vi "Extract CMD_Data.vi"(11 "Frame":string) -> (1 "DATA":string, 2 "Status":string, 3 "CMD":string)   [LabVIEW 2020, in "Library Test.lvlib" / "P2056_Send_Command_UART.lvclass"]
uses:
  P2056_Send_Command_UART.lvclass
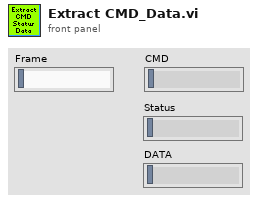
[diagram p1: front panel]
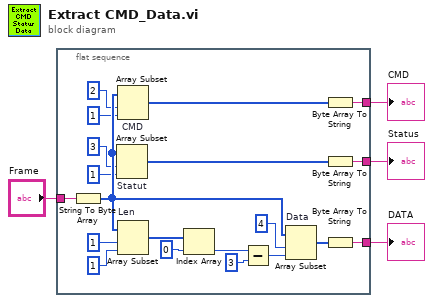
[diagram p0: block diagram]
diagram:
  n1 = flat-sequence {
    tunnel: "Frame" -> [w9]
    tunnel: [w8] -> w4
    tunnel: [w7] -> w3
    tunnel: [w5] -> w1
    frame #0 {
      n2 = String To Byte Array(string=w9) -> (unsigned byte array=w22:u8[])
      n3 = Array Subset "Statut"(array=w22, index=3 ("indice"), length=1 ("longueur")) -> (w6:u8[])
      n4 = Array Subset "CMD"(array=w22, index=2 ("indice"), length=1 ("longueur")) -> (w12:u8[])
      n5 = Array Subset "Len"(array=w22, index=1 ("indice"), length=1 ("longueur")) -> (w23:u8[])
      n6 = Index Array(array=w23, index=0 ("indice")) -> (element=w24:u8)
      n7 = Subtract(x=w24, y=u8 3) -> (x-y=w11:u8)
      n8 = Array Subset "Data"(array=w22, index=4 ("indice"), length=w11) -> (w10:u8[])
      n9 = Byte Array To String(unsigned byte array=w12) -> (string=w7:string)
      n10 = Byte Array To String(unsigned byte array=w6) -> (string=w5:string)
      n11 = Byte Array To String(unsigned byte array=w10) -> (string=w8:string)
    }
  }
  "DATA" <- w4
  "CMD" <- w3
  "Status" <- w1
